vi "sem_timedwait.vi"(8 "error in (no error)":errorcluster, 10 "absolute timeout":cluster{"sec":u64, "nsec":u64}, 11 "sempahore ptr in":u64) -> (0 "error out":errorcluster, 2 "timed out?":bool, 3 "semaphore ptr out":u64)   [LabVIEW 2013, in "Linux RT IPC.POSIX Threads.lvlib" / "POSIX Thread Object.lvclass"]
uses:
  POSIX Thread Object.lvclass
  Controls/pthread functions.ctl
  <vilib>/NI/NI Linux RT Errno/Controls/Public/errno.ctl
  <vilib>/NI/NI Linux RT Errno/Linux Errno.lvlib
  <vilib>/NI/NI Linux RT Utilities/Linux RT Utilities.lvlib
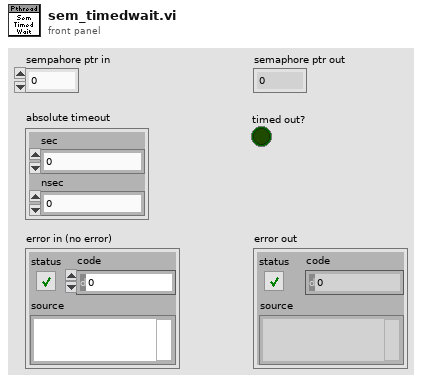
[diagram p1: front panel]
types:
  T1 = typedef "Linux Errno.lvlib/errno.ctl" = enum16{"NO ERROR", "EPERM", "ENOENT", "ESRCH", "EINTR", "EIO", "ENXIO", "E2BIG", "ENOEXEC", "EBADF", "ECHILD", "EAGAIN", "ENOMEM", "EACCES", "EFAULT", "ENOTBLK", "EBUSY", "EEXIST", "EXDEV", "ENODEV", "ENOTDIR", "EISDIR", "EINVAL", "ENFILE", "EMFILE", "ENOTTY", "ETXTBSY", "EFBIG", "ENOSPC", "ESPIPE", "EROFS", "EMLINK", "EPIPE", "EDOM", "ERANGE", "EDADLK", "ENAMETOOLONG", "ENOLCK", "ENOSYS", "ENOTEMPTY", "ELOOP", "EWOULDBLOCK", "ENOMSG", "EIDRM", "ECHRNG", "EL2NSYNC", "EL3HLT", "EL3RST", "ELNRNG", "EUNATCH", "ENOCSI", "EL2HLT", "EBADE", "EBADR", "EXFULL", "ENOANO", "EBADRQC", "EBADSLT", "EDEADLOCK", "EBFONT", "ENOSTR", "ENODATA", "ETIME", "ENOSR", "ENONET", "ENOPKG", "EREMOTE", "ENOLINK", "EADV", "ESRMNT", "ECOMM", "EPROTO", "EMULTIHOP", "EDOTDOT", "EBADMSG", "EOVERFLOW", "ENOTUNIQ", "EBADFD", "EREMCHG", "ELIBACC", "ELIBBAD", "ELIBSCN", "ELIBMAX", "ELIBEXEC", "ELISEQ", "ERESTART", "ESTRPIPE", "EUSERS", "ENOTSOCK", "EDESTADDRREQ", "EMSGSIZE", "EPROTOTYPE", "ENOPROTOOPT", "EPROTONOSUPPORT", "ESOCKTNOSUPPORT", "EOPNOTSUPP", "EPFNOSUPPORT", "EAFNOSUPPORT", "EADDRINUSE", "EADDRNOTAVAIL", "ENETDOWN", "ENETUNREACH", "ENETRESET", "ECONNABORTED", "ECONNRESET", "ENOBUFS", "EISCONN", "ENOTCONN", "ESHUTDOWN", "ETOOMANYREFS", "ETIMEDOUT", "ECONNREFUSED", "EHOSTDOWN", "EHOSTUNREACH", "EALREADY", "EINPROGRESS", "ESTALE", "EUCLEAN", "ENOTNAM", "ENAVAIL", "EISNAM", "EREMOTEIO", "EDQUOT", "ENOMEDIUM", "EMEDIUMTYPE", "ECANCELED", "ENOKEY", "EKEYEXPIRED", "EKEYREVOKED", "EKEYREJECTED", "EOWNERDEAD", "ENOTRECOVERABLE", "ERFKILL", "EHWPOISON", "UNDEFINED"}
  T2 = typedef "Linux RT IPC.POSIX Threads.lvlib/POSIX Thread Object.lvclass/pthread functions.ctl" = enum16{"unspecified", "pthread_condattr_init", "pthread_condattr_destroy", "pthread_condattr_getclock", "pthread_condattr_setclock", "pthread_condattr_getpshared", "pthread_condattr_setpshared", "pthread_cond_init", "pthread_cond_destroy", "pthread_cond_broadcast", "pthread_cond_signal", "pthread_cond_timedwait", "pthread_cond_wait", "pthread_mutexattr_init", "pthread_mutexattr_destroy", "pthread_mutexattr_getprioceiling", "pthread_mutexattr_setprioceiling", "pthread_mutexattr_getprotocol", "pthread_mutexattr_setprotocol", "pthread_mutexattr_getpshared", "pthread_mutexattr_setpshared", "pthread_mutexattr_gettype", "pthread_mutexattr_settype", "pthread_mutex_init", "pthread_mutex_destroy", "pthread_mutex_getprioceiling", "pthread_mutex_setprioceiling", "pthread_mutex_lock", "pthread_mutex_timedlock", "pthread_mutex_trylock", "pthread_mutex_unlock", "sem_destroy", "sem_getvalue", "sem_init", "sem_post", "sem_timedwait", "sem_trywait", "sem_wait", "barrier_init", "barrier_destroy", "barrier_wait", "barrierattr_init", "barrierattr_destroy", "barrierattr_getpshared", "barrierattr_setpshared"}
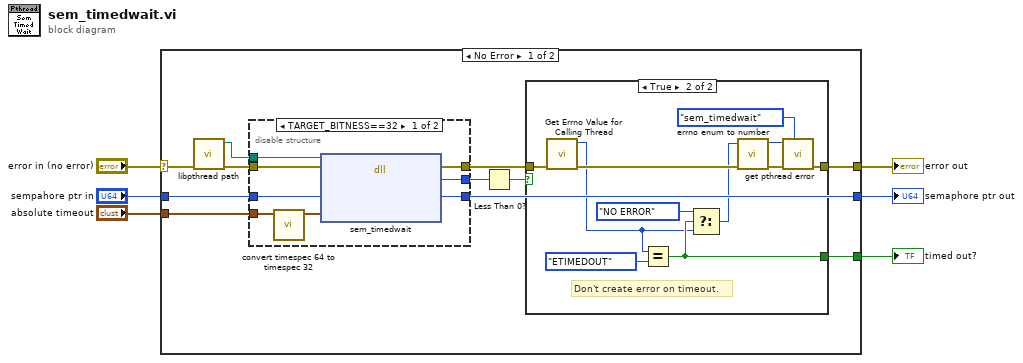
[diagram p0: block diagram]
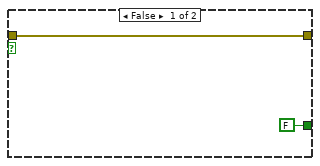
[diagram p2: hidden frame]
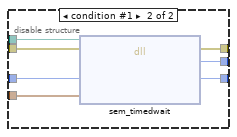
[diagram p3: hidden frame]
diagram:
  n1 = case shown="No Error" "error in (no error)" {
    selector: "error in (no error)" -> [w17 w47]
    tunnel: "sempahore ptr in" -> [w13 w46]
    tunnel: [w16 w47] -> w4
    tunnel: [w9 w46] -> w3
    tunnel: "absolute timeout" -> [w12 _]
    tunnel: [w8 _] -> w1
    frame No Error {
      n2 = call "libpthread path.vi"("error in (no error)"=w17) -> ("error out"=w15:errorcluster, "path to libpthread"=w14:path)  [unwired: 9 in]
      n3 = disable-structure shown="TARGET_BITNESS==32" {
        disable-tunnel: w15 -> [w36 w44]
        disable-tunnel: [w35 w43] -> w11
        disable-tunnel: [w33 w41] -> w9
        disable-tunnel: [w34 w42] -> w10
        disable-tunnel: w13 -> [w32 w40]
        disable-tunnel: w14 -> [w37 w45]
        disable-tunnel: w12 -> [w38 w39]
        frame condition #0 (active) {
          n4 = call <vilib>:"convert timespec 64 to timespec 32.vi"("timespec 64"=w38) -> ("timespec 32"=w31:cluster{"sec":u32, "nsec":u32})  [unwired: 10 in]
          n5 = dll-call lib="?" fn="sem_timedwait"(path in=w37, error in=w36, "sem"=w32, "absolute timeout"=w31) -> (error out=w35:errorcluster, "errno"=w34:i32, "sem"=w33:u64)  [unwired: 2 in, 1 out]
        }
        frame condition #1 {
          n6 = dll-call lib="?" fn="sem_timedwait"(path in=w45, error in=w44, "sem"=w40, "absolute timeout"=w39) -> (error out=w43:errorcluster, "errno"=w42:i32, "sem"=w41:u64)  [unwired: 2 in, 1 out]
        }
      }
      n7 = Less Than 0?(x=w10) -> (x < 0?=w7:bool)
      n8 = case shown="True" w7 {
        tunnel: [w18 w30] -> w16
        tunnel: w11 -> [w18 w28]
        tunnel: [FALSE w21] -> w8
        frame False {
        }
        frame True {
          # "Don't create error on timeout."
          n9 = call <vilib>:"Get Errno Value for Calling Thread.vi"("error in (no error)"=w28) -> ("error out"=w23:errorcluster, "errno"=w20:T1)  [unwired: 9 in]
          n10 = Equal?(x=w20, y=errno."ETIMEDOUT" ("errno")) -> (x = y?=w21:bool)
          n11 = Select(t=errno."NO ERROR" ("errno"), s=w21, f=w20) -> (s? t:f=w22:T1)
          n12 = call <vilib>:"errno enum to number.vi"("error in (no error)"=w23, "errno enum"=w22) -> ("error out"=w27:errorcluster, "errno number"=w26:i32)  [unwired: 8 in]
          n13 = call "get pthread error.vi"("function"=pthread_functions."sem_timedwait", "error in (no error)"=w27, "errno"=w26) -> ("error out"=w30:errorcluster)  [unwired: 8 in]
        }
      }
    }
    frame Error {
    }
  }
  "error out" <- w4
  "semaphore ptr out" <- w3
  "timed out?" <- w1
